vi "Main.vi"() -> ()   [LabVIEW 2023]
uses:
  UserCredentials.ctl
  Schedule.ctl
  stepvariables.ctl
  biasdiff.ctl
  gridvals.ctl
  remoterdgs.ctl
  QSM - Main/Controls/State Machine Message.ctl
  QSM - Main/Controls/Message Queue Element Position.ctl
  QSM - Main/QSM - Main.lvlib
panel:
  in  "Digital IO":bool[](array[boolean])
  in  "Analog IO":dbl[](array[numeric])
  in  "OffsetGain":dbl[](array[numeric])
  out "remrdgs":T1
  in  "Param Gx Only":cluster{"P06 G1 ONLY":bool, "P21 G2 ONLY":bool}
  in  "GXVALS":T2
  in  "BIAS DIFF":T3 {"DIFF" step=10.0; "BIAS" step=10.0}
  out "LIMITS":sgl[](array[numeric])
  out "Run Results":i32[](listbox)
  out "ALARM":bool
  out "PROC NOK":bool
  in  "ALARMS":bool[](array[boolean])=[FALSE]
  in  "PROC OK":bool[](array[boolean])=[TRUE]
  out "STEP VARS":T4
  in  "PLC CURRENT STEP":u16
  in  "RESET Button":bool
  in  "RUN Button":bool
  in  "FINAL STEP":u16
  out "CURRENT STEP":u16
  in  "FIRST STEP":u16
  in  "ALARMS BUtton":bool
  in  "LIMITS Button":bool
  in  "IO/DOCS Button":bool
  in  "ENTER OP":string
  in  "ENTER SN":string
  in  "View Sched Button":bool
  in  "Schedule":T5 caption="Multicolumn Listbox"
  out "SchedNames[]":string[](array[string])
  out "SchedName":string
  out "SchedNum":string
  in  "sched sel Button":bool
  out "schd61-80":u32
  out "schd31-60":u32
  out "schd1-30":u32
  out "AP%":dbl
  out "T10":dbl
  out "T100":dbl
  out "HS":dbl
  out "RTC":dbl
  out "NAME":string
  out "TUBE":dbl
  in  "Load Tube Button":bool
  in  "Error In":errorcluster
  out "Error Out":errorcluster
  in  "Security Button":bool
  in  "stop":bool
  out "Access":u16
  out "Op Name":string
  out "BADGE NUMBER":string
  in  "Log In Button":bool
  in  "Editor Button":bool
  in  "User Creds":T6
  # "--STEP VARIABLES--"
  # "--GRID TANK VALUES--"
  # "--CONTROLS--"
  # "ENTER SN"
  # "ENTER OP"
  # "--READINGS--"
  # "FOCAL SPOT GRID TANK RUN RESULTS"
  # "OFFSET"
  # "GAIN"
  # "OFFSET"
  # "GAIN"
  # "GAIN"
  # "OFFSET"
  # "GAIN"
  # "STEP"
  # "NAME"
  # "NOTES"
  # "PARAMS"
  # "KV SP"
  # "KV RDG"
  # "MA/IF SP"
  # "MA/IF RDG"
  # "EXP sec SP"
  # "EXP sec RDG"
  # "COOL sec SP"
  # "COOL sec RDG"
  # "scans.Mode"
  # "data item"
  # "min"
  # "max"
  # "init BIAS SP"
  # "init BIAS RDG"
  # "init DIFF SP"
  # "max Gx"
  # "init EfDr SP"
  # "init EfDr RDG"
  # "max Tries"
  # "TEST"
  # "LIM1"
  # "LIM2"
  # "LIM4"
  # "LIM3"
  # "CHAIN SCHEDS"
  # "RPTS"
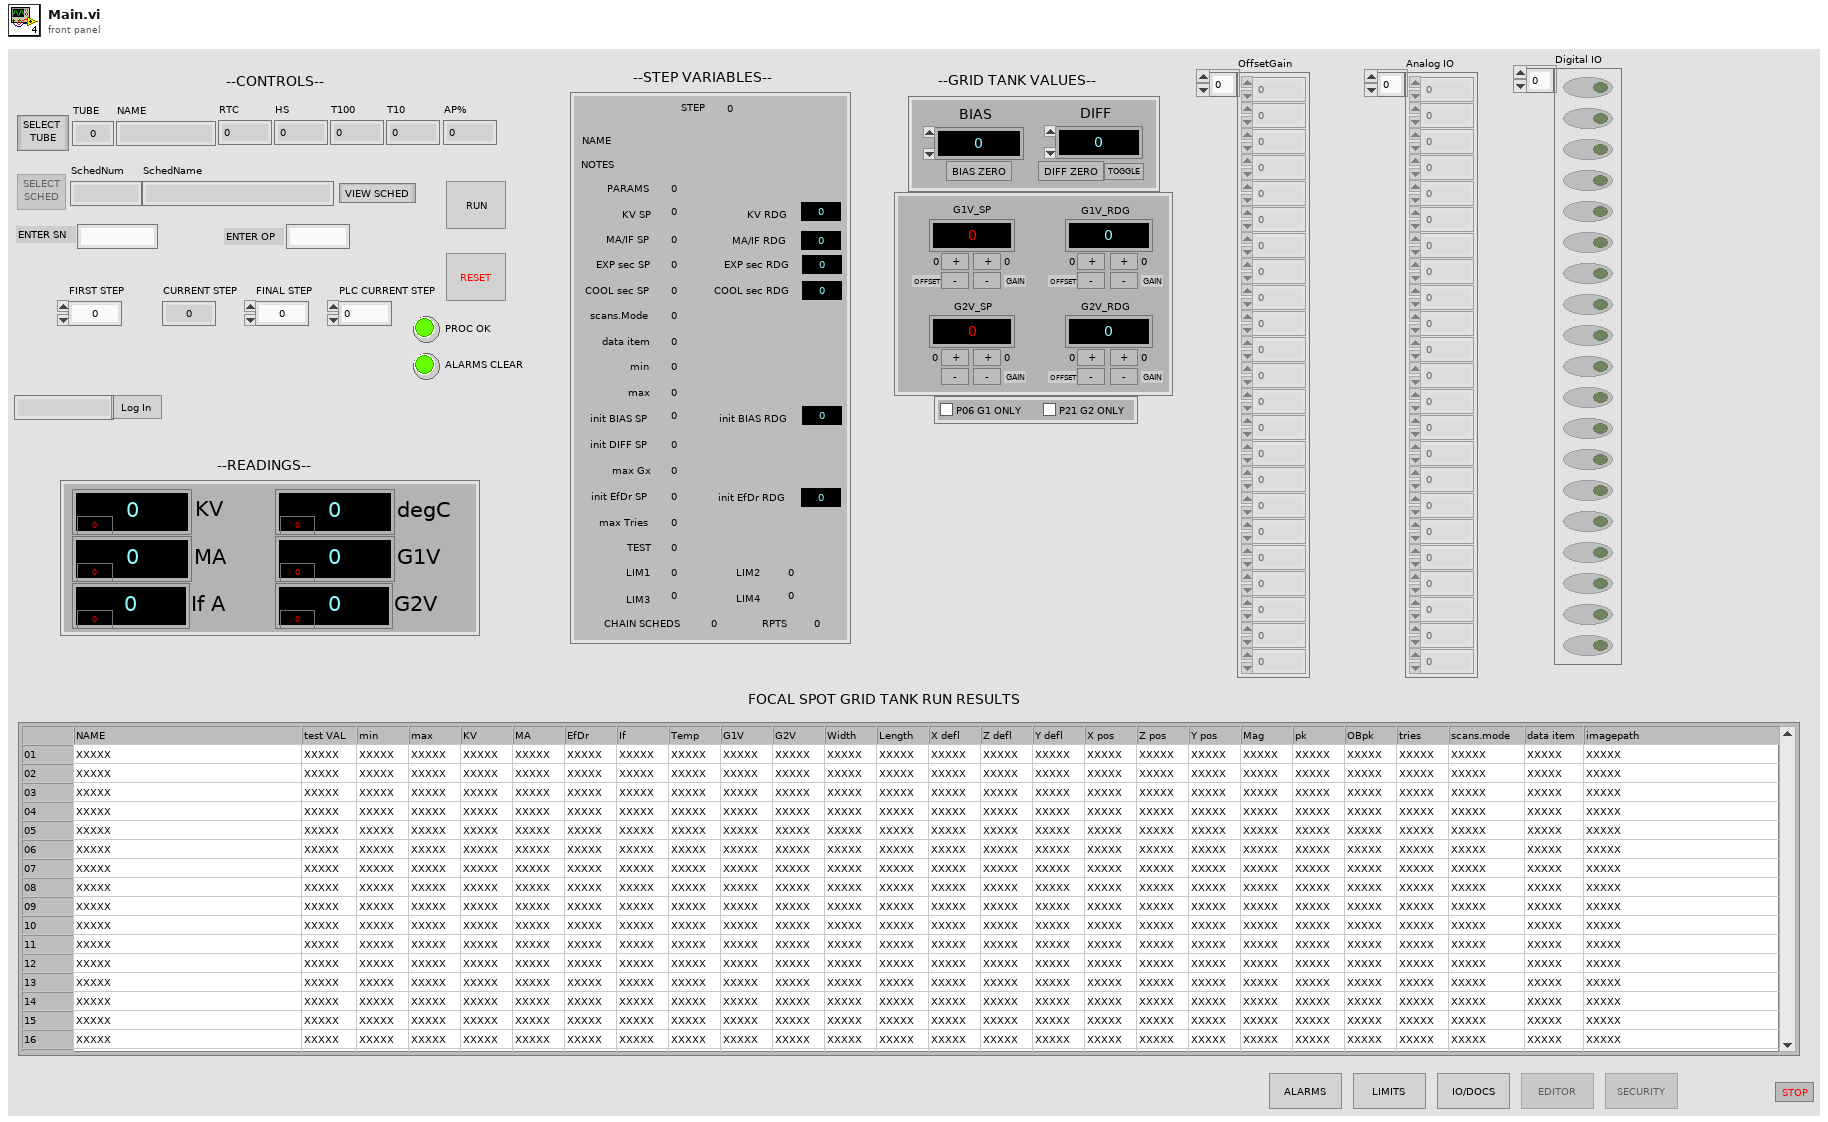
[diagram p1: front panel]
types:
  T1 = typedef "remoterdgs.ctl" = cluster{"remKVrdg":dbl, "remMArdg":dbl, "remIfArdg":dbl, "Temprdg":dbl, "G1Vrdg":dbl, "G2Vrdg":dbl, "remKVsp":dbl, "remMAsp":dbl, "remIfAsp":dbl, "Tempsp":dbl, "G1Vsp":dbl, "G2Vsp":dbl}
  T2 = typedef "gridvals.ctl" = cluster{"G1V_SP":dbl, "G2V_SP":dbl, "G1V_RDG":dbl, "G2V_RDG":dbl, "G1sp offset up":bool, "G1sp offset down":bool, "G1sp gain up":bool, "G1sp gain down":bool, "G1rdg offset up":bool, "G1rdg offset down":bool, "G1rdg gain up":bool, "G1rdg gain down":bool, "G2sp offset up":bool, "G2sp offset down":bool, "G2sp gain up":bool, "G2sp gain down":bool, "G2rdg offset up":bool, "G2rdg offset down":bool, "G2rdg gain up":bool, "G2rdg gain down":bool, "g1spoffset":dbl, "g1spgain":dbl, "g2spoffset":dbl, "g2spgain":dbl, "g1rdgoffset":dbl, "g1rdggain":dbl, "g2rdgoffset":dbl, "g2rdggain":dbl}
  T3 = typedef "biasdiff.ctl" = cluster{"BIAS":dbl, "BIAS_ZER":bool, "BIAS_ZER 2":bool, "DIFF_TOGGLE":bool, "DIFF":dbl}
  T4 = typedef "stepvariables.ctl" = cluster{"NAME":string, "NOTES":string, "PARAMS":u32, "KV  SP":dbl, "KV  RDG":dbl, "MA/IF  SP":dbl, "MA/IF  RDG":dbl, "init BIAS SP":dbl, "init BIAS RDG":dbl, "max Gx":dbl, "TEST":u32, "min":dbl, "max":dbl, "LIM1":dbl, "LIM2":dbl, "LIM3":dbl, "LIM4":dbl, "data item":dbl, "chain scheds":dbl, "REPEATS":dbl, "STEP NUM":u32, "EXP s SP":dbl, "EXP s RDG":dbl, "COOL s SP":dbl, "COOL s RDG":dbl, "scans mode":dbl, "init EfDr":dbl, "init EfDr RDG":dbl, "max Tries":dbl, "init DIFF SP":dbl}
  T5 = typedef "Schedule.ctl" = i32
  T6 = typedef "UserCredentials.ctl" = cluster{"Badge Number":string, "Name":string, "Access":enum16{"", "Operator", "Admin", "Engineer"}}
  T7 = typedef "QSM - Main.lvlib/State Machine Message.ctl" = enum16{"Initialize", "Operator Signon", "Editor", "Security", "Select Tube", "Select Sched", "View Sched", "View IO/DOCS", "View LIMITS", "View ALARMS", "Start Step Change", "New Serial Number", "RUN Initiated", "RESET Initiated", "PLC Step Change", "PROC OK CHECK", "PROC NOK", "ALARM CHECK", "ALARM ACTIVE", "Handle Error", "Exit"}
  T8 = typedef "QSM - Main.lvlib/Message Queue Element Position.ctl" = enum16{"Front", "Back"}
  T9 = enum8{"Enabled", "Disabled", "Disabled and Grayed Out"}
  T10 = typedef "UserCredentials.ctl" = cluster{"Badge Number":string, "Name":string, "Access":u16}
  T11 = cluster{"NO GRID TANK":bool, "NO GRID TANK 2":bool, "NO GRID TANK 3":bool, "NO GRID TANK 4":bool, "NO GRID TANK 5":bool, "NO GRID TANK 6":bool, "NO GRID TANK 7":bool, "NO GRID TANK 8":bool}
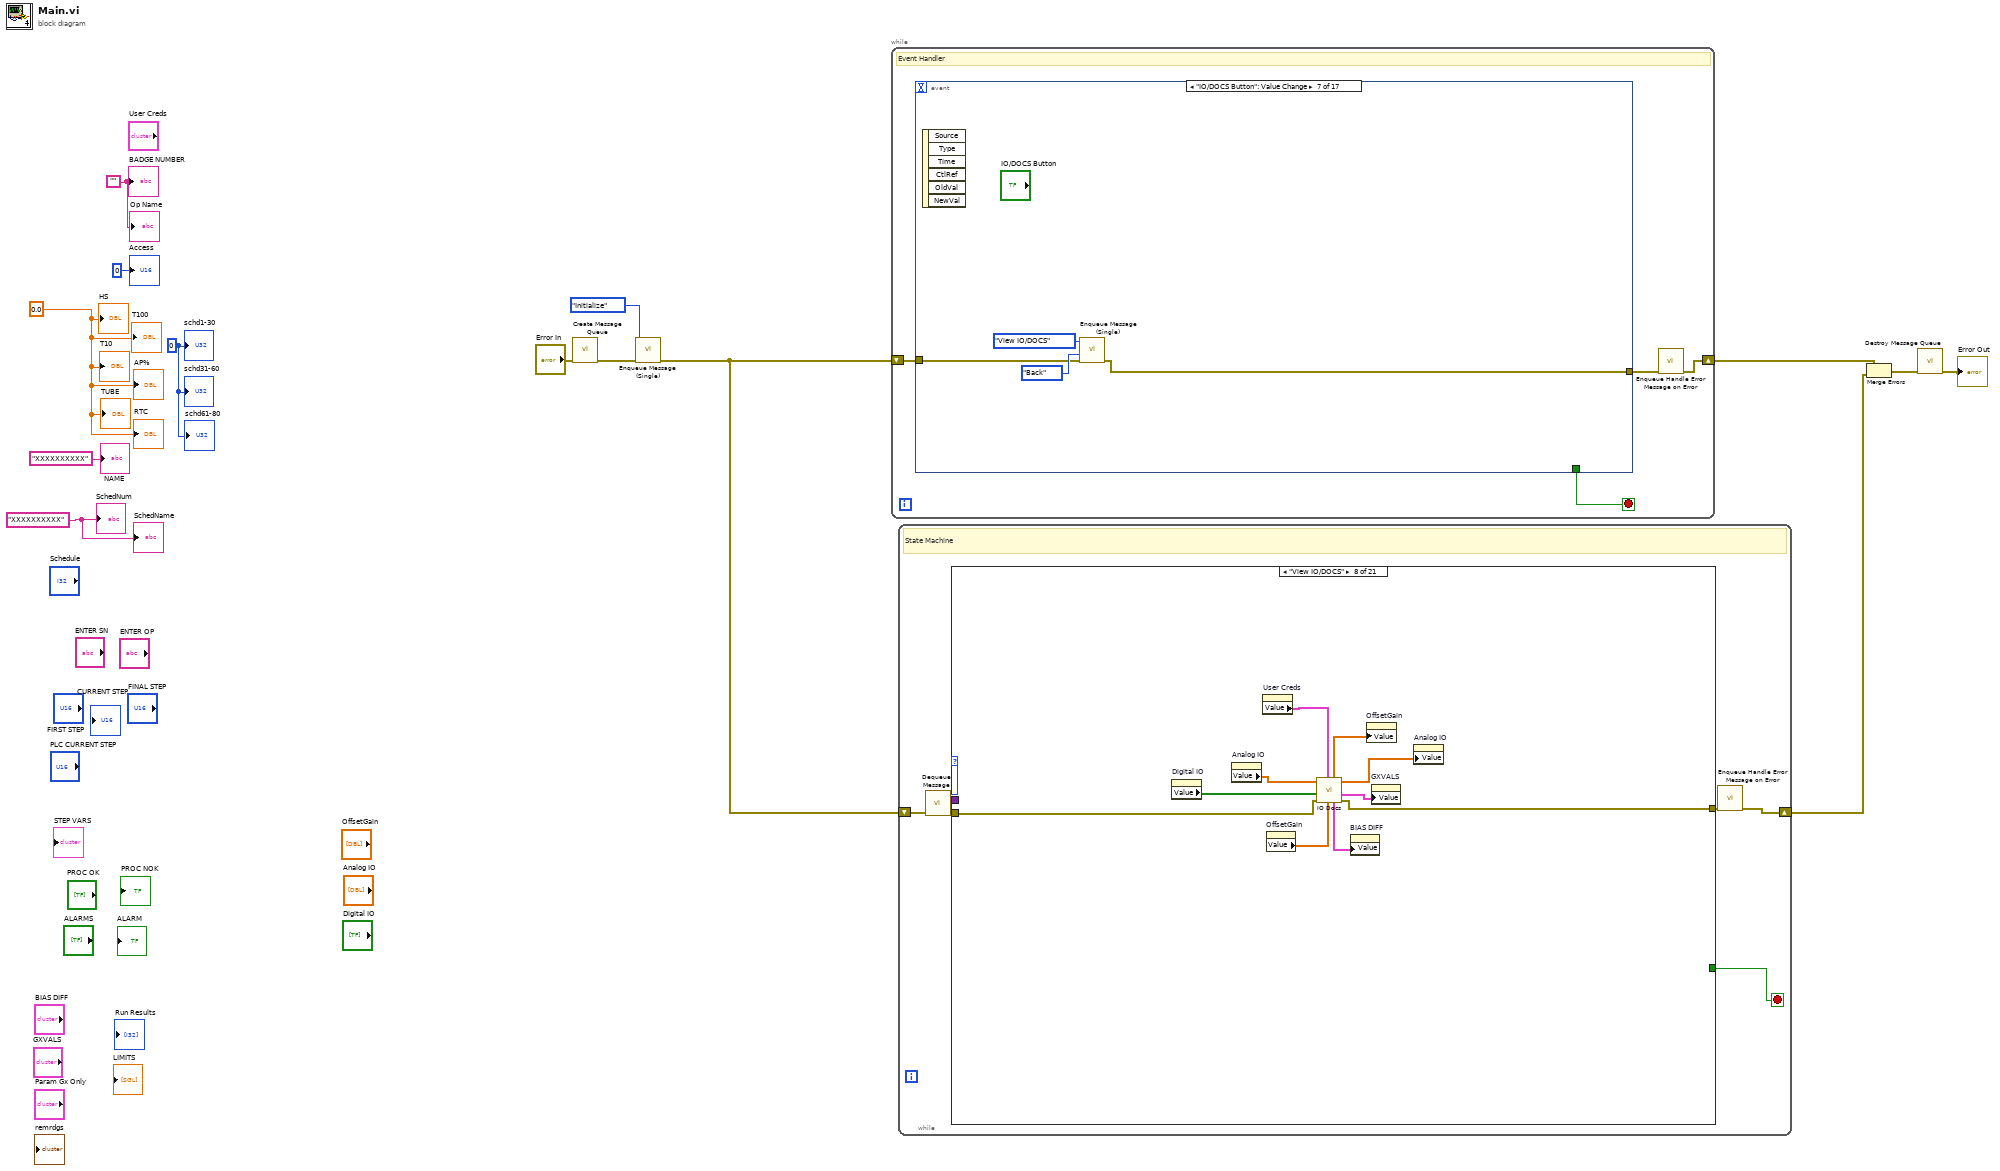
[diagram p0: block diagram]
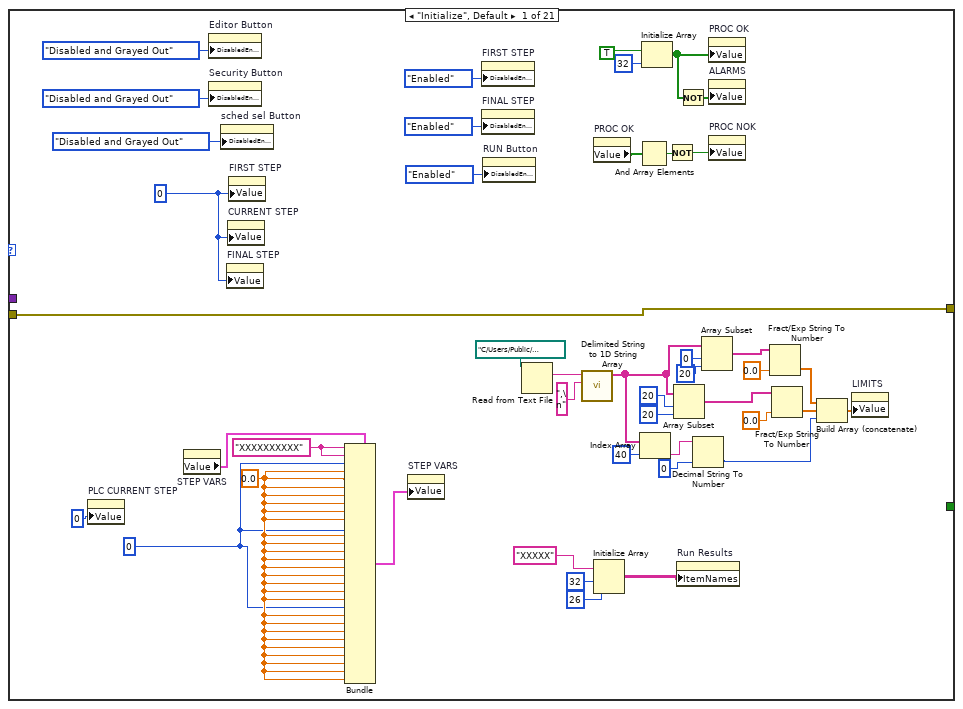
[diagram p2: hidden frame]
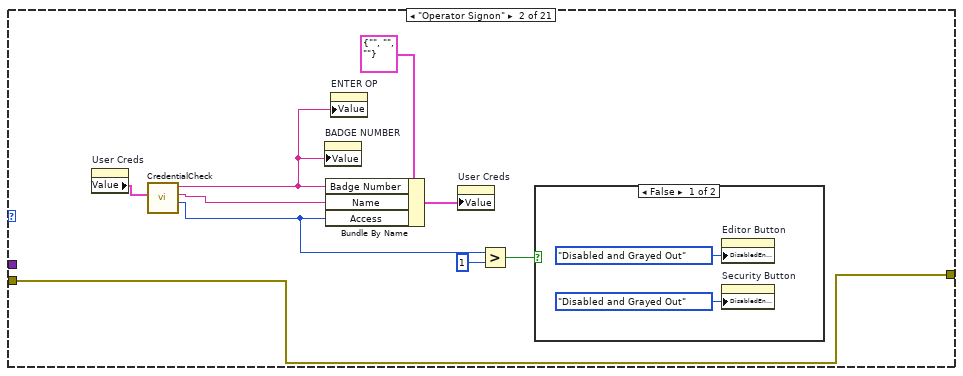
[diagram p3: hidden frame]
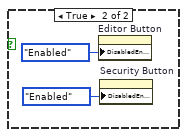
[diagram p4: hidden frame]
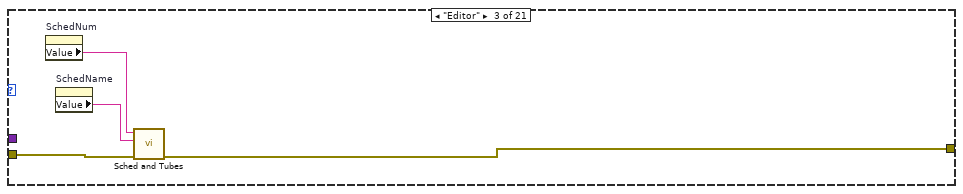
[diagram p5: hidden frame]
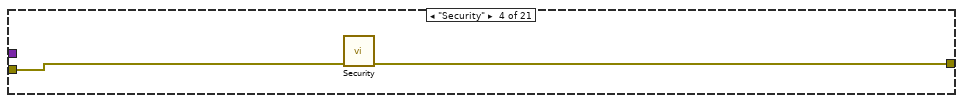
[diagram p6: hidden frame]
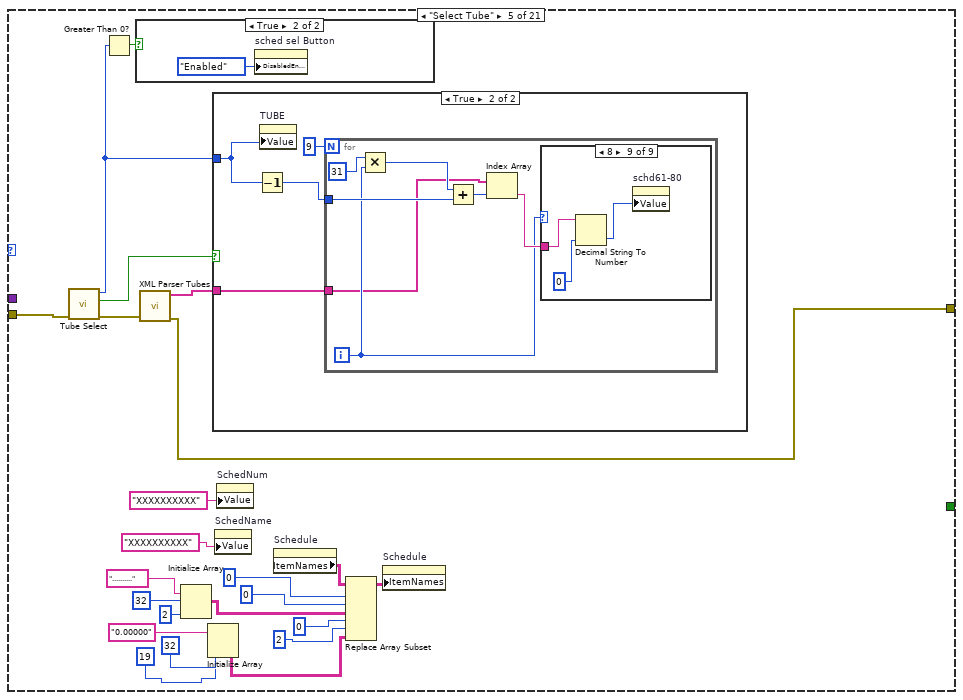
[diagram p7: hidden frame]
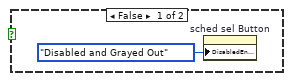
[diagram p8: hidden frame]
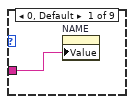
[diagram p10: hidden frame]
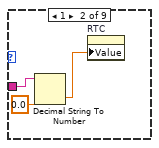
[diagram p11: hidden frame]
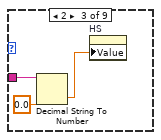
[diagram p12: hidden frame]
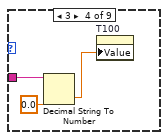
[diagram p13: hidden frame]
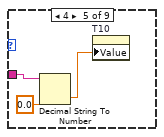
[diagram p14: hidden frame]
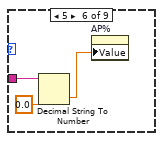
[diagram p15: hidden frame]
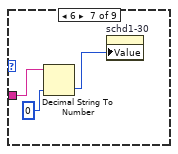
[diagram p16: hidden frame]
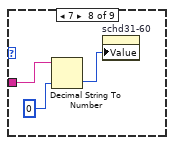
[diagram p17: hidden frame]
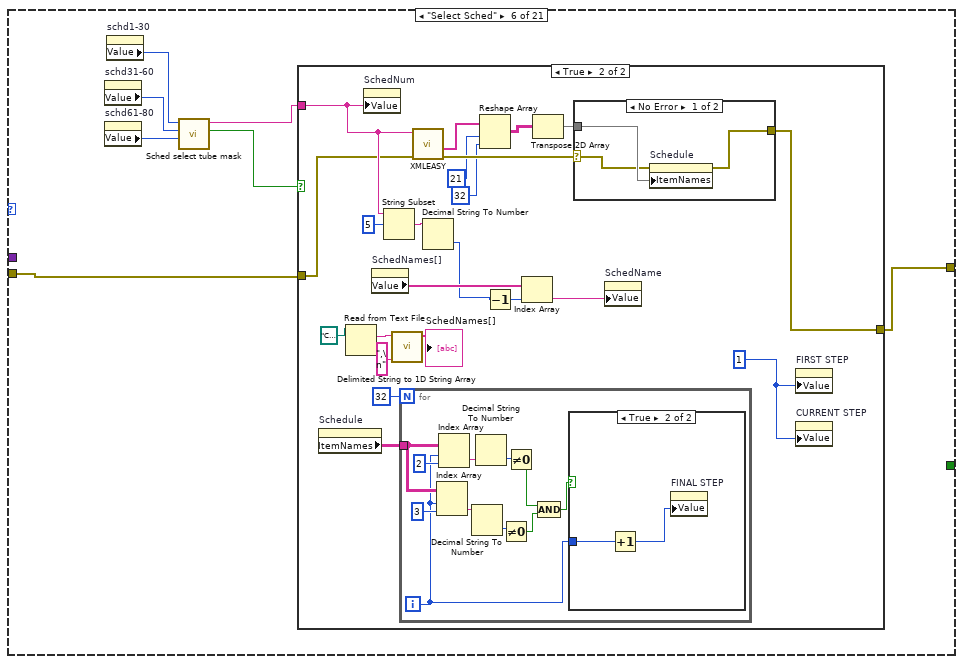
[diagram p18: hidden frame]
diagram:
  w1 = "XXXXXXXXXX" ("SchedNum")
  w2 = u32 0 ("schd1-30")
  w3 = 0.0 ("HS")
  w14 = "" ("Badge Number")
  n1 = call "Create Message Queue.vi"("Error In"="Error In") -> ("Error Out"=w12:errorcluster)  [unwired: 10 in]
  n2 = call "Enqueue Message (Single).vi"("Error In"=w12, "State Machine Message"=State_Machine_Message."Initialize") -> ("Error Out"=w6:errorcluster)  [unwired: 9 in]
  n3 = while {
    shift-right: [w15] -> w10
    shift-left: w6 -> [w17]
    stop <- w18 stop-if-true
    # "Event Handler"
    n4 = event shown="[6] \"IO/DOCS Button\": Value Change" {
      selector: _ -> [_ _ _ _ _ _ _ _ _ _ _ _ _ _ _ _ _]
      dyn-events: _ -> [_ _ _ _ _ _ _ _ _ _ _ _ _ _ _ _ _]
      timeout: _ -> [_ _ _ _ _ _ _ _ _ _ _ _ _ _ _ _ _]
      tunnel: [_ _ _ _ _ _ _ _ _ _ _ _ _ _ _ _ TRUE] -> w18
      tunnel: w17 -> [w20 w24 w30 w32 w36 w40 w44 w48 w52 w56 w60 w64 w68 w72 w76 w80 w84]
      tunnel: [w19 w23 w29 w31 w35 w39 w43 w47 w51 w55 w59 w63 w67 w71 w75 w79 w83] -> w16
      event "Log In Button": Value Change {
        n5 = event-data() -> ()  [unwired: 1 in, 6 out]
        n6 = call "Enqueue Message (Single).vi"("Error In"=w20, "Message Position"=Message_Queue_Element_Position."Back", "State Machine Message"=State_Machine_Message."Operator Signon") -> ("Error Out"=w19:errorcluster)  [unwired: 8 in]
      }
      event "Editor Button": Value Change {
        n7 = event-data() -> ()  [unwired: 1 in, 6 out]
        n8 = call "Enqueue Message (Single).vi"("Error In"=w24, "Message Position"=Message_Queue_Element_Position."Back", "State Machine Message"=State_Machine_Message."Editor") -> ("Error Out"=w23:errorcluster)  [unwired: 8 in]
      }
      event "Security Button": Value Change {
        n9 = event-data() -> ()  [unwired: 1 in, 6 out]
        n10 = call "Enqueue Message (Single).vi"("Error In"=w30, "Message Position"=Message_Queue_Element_Position."Back", "State Machine Message"=State_Machine_Message."Security") -> ("Error Out"=w29:errorcluster)  [unwired: 8 in]
      }
      event "Load Tube Button": Value Change {
        n11 = event-data() -> ()  [unwired: 1 in, 6 out]
        n12 = call "Enqueue Message (Single).vi"("Error In"=w32, "Message Position"=Message_Queue_Element_Position."Back", "State Machine Message"=State_Machine_Message."Select Tube") -> ("Error Out"=w31:errorcluster)  [unwired: 8 in]
      }
      event "sched sel Button": Value Change {
        n13 = event-data() -> ()  [unwired: 1 in, 6 out]
        n14 = call "Enqueue Message (Single).vi"("Error In"=w36, "Message Position"=Message_Queue_Element_Position."Back", "State Machine Message"=State_Machine_Message."Select Sched") -> ("Error Out"=w35:errorcluster)  [unwired: 8 in]
      }
      event "View Sched Button": Value Change {
        n15 = event-data() -> ()  [unwired: 1 in, 6 out]
        n16 = call "Enqueue Message (Single).vi"("Error In"=w40, "Message Position"=Message_Queue_Element_Position."Back", "State Machine Message"=State_Machine_Message."View Sched") -> ("Error Out"=w39:errorcluster)  [unwired: 8 in]
      }
      event "IO/DOCS Button": Value Change {
        n17 = event-data() -> ()  [unwired: 1 in, 6 out]
        n18 = call "Enqueue Message (Single).vi"("Error In"=w44, "Message Position"=Message_Queue_Element_Position."Back", "State Machine Message"=State_Machine_Message."View IO/DOCS") -> ("Error Out"=w43:errorcluster)  [unwired: 8 in]
      }
      event "LIMITS Button": Value Change {
        n19 = event-data() -> ()  [unwired: 1 in, 6 out]
        n20 = call "Enqueue Message (Single).vi"("Error In"=w48, "Message Position"=Message_Queue_Element_Position."Back", "State Machine Message"=State_Machine_Message."View LIMITS") -> ("Error Out"=w47:errorcluster)  [unwired: 8 in]
      }
      event "ALARMS BUtton": Value Change {
        n21 = event-data() -> ()  [unwired: 1 in, 6 out]
        n22 = call "Enqueue Message (Single).vi"("Error In"=w52, "Message Position"=Message_Queue_Element_Position."Back", "State Machine Message"=State_Machine_Message."View ALARMS") -> ("Error Out"=w51:errorcluster)  [unwired: 8 in]
      }
      event "FIRST STEP": Value Change {
        n23 = event-data() -> ()  [unwired: 1 in, 6 out]
        n24 = call "Enqueue Message (Single).vi"("Error In"=w56, "Message Position"=Message_Queue_Element_Position."Back", "State Machine Message"=State_Machine_Message."Start Step Change") -> ("Error Out"=w55:errorcluster)  [unwired: 8 in]
      }
      event "PLC CURRENT STEP": Value Change {
        n25 = event-data() -> ()  [unwired: 1 in, 6 out]
        n26 = call "Enqueue Message (Single).vi"("Error In"=w60, "Message Position"=Message_Queue_Element_Position."Back", "State Machine Message"=State_Machine_Message."PLC Step Change") -> ("Error Out"=w59:errorcluster)  [unwired: 8 in]
      }
      event "ENTER SN": Value Change {
        n27 = event-data() -> ()  [unwired: 1 in, 6 out]
        n28 = call "Enqueue Message (Single).vi"("Error In"=w64, "Message Position"=Message_Queue_Element_Position."Back", "State Machine Message"=State_Machine_Message."PLC Step Change") -> ("Error Out"=w63:errorcluster)  [unwired: 8 in]
      }
      event "RUN Button": Value Change {
        n29 = event-data() -> ()  [unwired: 1 in, 6 out]
        n30 = call "Enqueue Message (Single).vi"("Error In"=w68, "Message Position"=Message_Queue_Element_Position."Back", "State Machine Message"=State_Machine_Message."RUN Initiated") -> ("Error Out"=w67:errorcluster)  [unwired: 8 in]
      }
      event "RESET Button": Value Change {
        n31 = event-data() -> ()  [unwired: 1 in, 6 out]
        n32 = call "Enqueue Message (Single).vi"("Error In"=w72, "Message Position"=Message_Queue_Element_Position."Back", "State Machine Message"=State_Machine_Message."RESET Initiated") -> ("Error Out"=w71:errorcluster)  [unwired: 8 in]
      }
      event "PROC OK": Value Change {
        n33 = event-data() -> ()  [unwired: 1 in, 6 out]
        n34 = call "Enqueue Message (Single).vi"("Error In"=w76, "Message Position"=Message_Queue_Element_Position."Front", "State Machine Message"=State_Machine_Message."PROC OK CHECK") -> ("Error Out"=w75:errorcluster)  [unwired: 8 in]
      }
      event "ALARMS": Value Change {
        n35 = event-data() -> ()  [unwired: 1 in, 6 out]
        n36 = call "Enqueue Message (Single).vi"("Error In"=w80, "Message Position"=Message_Queue_Element_Position."Front", "State Machine Message"=State_Machine_Message."ALARM CHECK") -> ("Error Out"=w79:errorcluster)  [unwired: 8 in]
      }
      event "stop": Value Change {
        n37 = event-data() -> ()  [unwired: 1 in, 6 out]
        n38 = call "Enqueue Message (Single).vi"("Error In"=w84, "Message Position"=Message_Queue_Element_Position."Front", "State Machine Message"=State_Machine_Message."Exit") -> ("Error Out"=w83:errorcluster)  [unwired: 8 in]
      }
    }
    n39 = call "Enqueue Handle Error Message on Error.vi"("Error In"=w16) -> ("Error Out"=w15:errorcluster)  [unwired: 10 in]
  }
  n40 = while {
    shift-right: [w90] -> w9
    shift-left: w6 -> [w88]
    stop <- w89 stop-if-true
    # "State Machine"
    n41 = call "Dequeue Message.vi"("Error In"=w88) -> ("Error Out"=w92:errorcluster, "Data"=w93:variant, "State Machine Message"=w94:T7)  [unwired: 8 in]
    n42 = case shown="\"View IO/DOCS\"" w94 {
      tunnel: w93 -> [_ _ _ _ _ _ _ _ _ _ _ _ _ _ _ _ _ _ _ w371 _]
      tunnel: w92 -> [w115 w141 w155 w157 w180 w220 w269 w279 w288 w297 w300 w302 w304 w332 w338 w344 w355 w358 w366 w369 w374]
      tunnel: [w115 w141 w154 w156 w176 w219 w269 w278 w287 w296 w298 w302 w304 w332 w338 w343 w355 w357 w366 w367 w373] -> w91
      tunnel: [_ _ _ _ _ _ _ _ _ _ _ _ _ _ _ _ _ _ _ _ TRUE] -> w89
      frame "Initialize", Default {
        w95 = u32 0 ("PARAMS")
        w130 = 0.0
        w131 = "XXXXXXXXXX" ("NAME")
        w135 = 0 ("STARTING STEP")
        n43 = property on="PLC CURRENT STEP" class="DigNum (strict)"("Value"=u16 0 ("PLC CURRENT STEP 2")) -> ()  [unwired: 2 in, 2 out]
        n44 = property on="STEP VARS" class="Clust (strict)"() -> ("Value"=w132:T4)  [unwired: 2 in, 2 out]
        n45 = property on="Editor Button" class="Bool"("DisabledEnum"=T9."Disabled and Grayed Out" ("Disabled")) -> ()  [unwired: 2 in, 2 out]
        n46 = property on="Security Button" class="Bool (strict)"("DisabledEnum"=T9."Disabled and Grayed Out" ("Disabled")) -> ()  [unwired: 2 in, 2 out]
        n47 = property on="sched sel Button" class="Bool (strict)"("DisabledEnum"=T9."Disabled and Grayed Out" ("Disabled")) -> ()  [unwired: 2 in, 2 out]
        n48 = property on="FINAL STEP" class="DigNum (strict)"("Value"=w135) -> ()  [unwired: 2 in, 2 out]
        n49 = property on="CURRENT STEP" class="DigNum (strict)"("Value"=w135) -> ()  [unwired: 2 in, 2 out]
        n50 = property on="FIRST STEP" class="DigNum (strict)"("Value"=w135) -> ()  [unwired: 2 in, 2 out]
        n51 = Bundle(cluster=w132, "NAME"=w131, "NOTES"=w131, "PARAMS"=w95, "KV  SP"=w130, "KV  RDG"=w130, "MA/IF  SP"=w130, "MA/IF  RDG"=w130, "init BIAS SP"=w130, "init BIAS RDG"=w130, "max Gx"=w130, "TEST"=w95, "min"=w130, "max"=w130, "LIM1"=w130, "LIM2"=w130, "LIM3"=w130, "LIM4"=w130, "data item"=w130, "chain scheds"=w130, "REPEATS"=w130, "STEP NUM"=w95, "EXP s SP"=w130, "EXP s RDG"=w130, "COOL s SP"=w130, "COOL s RDG"=w130, "scans mode"=w130, "init EfDr"=w130, "init EfDr RDG"=w130, "max Tries"=w130, "init DIFF SP"=w130) -> (w96:T4)
        n52 = property on="STEP VARS" class="Clust (strict)"("Value"=w96) -> ()  [unwired: 2 in, 2 out]
        n53 = property on="FIRST STEP" class="DigNum (strict)"("DisabledEnum"=T9."Enabled" ("Disabled")) -> ()  [unwired: 2 in, 2 out]
        n54 = property on="FINAL STEP" class="DigNum (strict)"("DisabledEnum"=T9."Enabled" ("Disabled")) -> ()  [unwired: 2 in, 2 out]
        n55 = property on="RUN Button" class="Bool (strict)"("DisabledEnum"=T9."Enabled" ("Disabled")) -> ()  [unwired: 2 in, 2 out]
        n56 = Read from Text File(file (use dialog)=path "C:/Users/Public/Documents/Grid2093/LIMITS/LIMITS.txt") -> (text=w110:string)  [unwired: 3 in, 3 out]
        n57 = call <vilib>:"Delimited String to 1D String Array.vi"("delimiter"=",\n", "delimited string"=w110) -> ("string array"=w113:string[])  [unwired: 9 in]
        n58 = property on="PROC OK" class="Arr (strict)"() -> ("Value"=w123:bool[])  [unwired: 2 in, 2 out]
        n59 = Initialize Array("XXXXX", 32 ("dimension size"), 26 ("dimension size")) -> (w117:string[][])
        n60 = And Array Elements(Boolean array=w123) -> (logical AND=w122:bool)
        n61 = Index Array(array=w113, index=40) -> (element=w114:string)
        n62 = Initialize Array(TRUE, 32 ("dimension size")) -> (w125:bool[])
        n63 = Not(x=w122) -> (.not. x?=w121:bool)
        n64 = Array Subset(array=w113, index=20, length=20) -> (w112:string[])
        n65 = property on="Run Results" class="MCListbox (strict)"("ItemNames"=w117) -> ()  [unwired: 2 in, 2 out]
        n66 = Not(x=w125) -> (.not. x?=w124:bool[])
        n67 = Decimal String To Number(string=w114, default (0L)=u32 0 ("default (0 I32)")) -> (number=w97:u32)  [unwired: 1 in, 1 out]
        n68 = Array Subset(array=w113, index=0, length=20) -> (w111:string[])
        n69 = property on="PROC OK" class="Arr (strict)"("Value"=w125) -> ()  [unwired: 2 in, 2 out]
        n70 = property on="ALARMS" class="Arr (strict)"("Value"=w124) -> ()  [unwired: 2 in, 2 out]
        n71 = property on="PROC NOK" class="Bool (strict)"("Value"=w121) -> ()  [unwired: 2 in, 2 out]
        n72 = Fract/Exp String To Number(string=w111, default (0 dbl)=sgl 0.0 ("default (0 DBL)")) -> (number=w99:sgl[])  [unwired: 2 in, 1 out]
        n73 = Fract/Exp String To Number(string=w112, default (0 dbl)=sgl 0.0 ("default (0 DBL)")) -> (number=w98:sgl[])  [unwired: 2 in, 1 out]
        n74 = Build Array (concatenate)(w99, w98, w97) -> (w116:sgl[])
        n75 = property on="LIMITS" class="Arr (strict)"("Value"=w116) -> ()  [unwired: 2 in, 2 out]
      }
      frame "Operator Signon" {
        n76 = property on="User Creds" class="Clust (strict)"() -> ("Value"=w139:T10)  [unwired: 2 in, 2 out]
        n77 = call "CredentialCheck.vi"("User Creds"=w139) -> ("Access"=w145:u16, "Name"=w144:string, "Badge Num"=w140:string)  [unwired: 8 in]
        n78 = property on="BADGE NUMBER" class="Str"("Value"=w140) -> ()  [unwired: 2 in, 2 out]
        n79 = Bundle By Name(cluster=T6 {"Badge Number"="", "Name"="", "Access"=enum.""} ("User Creds"), "Badge Number"=w140, "Name"=w144, "Access"=w145) -> (w143:T6)
        n80 = property on="ENTER OP" class="Str"("Value"=w140) -> ()  [unwired: 2 in, 2 out]
        n81 = property on="User Creds" class="Clust (strict)"("Value"=w143) -> ()  [unwired: 2 in, 2 out]
        n82 = Greater?(x=w145, y=u16 1) -> (0:w142:bool)
        n83 = case shown="False" w142 {
          frame False {
            n84 = property on="Editor Button" class="Bool"("DisabledEnum"=T9."Disabled and Grayed Out" ("Disabled")) -> ()  [unwired: 2 in, 2 out]
            n85 = property on="Security Button" class="Bool (strict)"("DisabledEnum"=T9."Disabled and Grayed Out" ("Disabled")) -> ()  [unwired: 2 in, 2 out]
          }
          frame True {
            n86 = property on="Editor Button" class="Bool"("DisabledEnum"=T9."Enabled" ("Disabled")) -> ()  [unwired: 2 in, 2 out]
            n87 = property on="Security Button" class="Bool (strict)"("DisabledEnum"=T9."Enabled" ("Disabled")) -> ()  [unwired: 2 in, 2 out]
          }
        }
      }
      frame "Editor" {
        n88 = property on="SchedNum" class="Str"() -> ("Value"=w153:string)  [unwired: 2 in, 2 out]
        n89 = property on="SchedName" class="Str"() -> ("Value"=w152:string)  [unwired: 2 in, 2 out]
        n90 = call "Sched and Tubes.vi"("Error In"=w155, "Preselected sched name"=w152, "Preselected sched"=w153) -> ("Error Out"=w154:errorcluster)  [unwired: 8 in]
      }
      frame "Security" {
        n91 = call "Security.vi"("Error In"=w157) -> ("error out"=w156:errorcluster)  [unwired: 10 in]
      }
      frame "Select Tube" {
        n92 = call "Tube Select.vi"("error in (no error)"=w180) -> ("error out"=w178:errorcluster, "Load"=w179:bool, "SelectedTube"=w175:i32)  [unwired: 7 in, 1 out]
        n93 = Greater Than 0?(x=w175) -> (x > 0?=w174:bool)
        n94 = case shown="True" w174 {
          frame False {
            n95 = property on="sched sel Button" class="Bool (strict)"("DisabledEnum"=T9."Disabled and Grayed Out" ("Disabled")) -> ()  [unwired: 2 in, 2 out]
          }
          frame True {
            n96 = property on="sched sel Button" class="Bool (strict)"("DisabledEnum"=T9."Enabled" ("Disabled")) -> ()  [unwired: 2 in, 2 out]
          }
        }
        n97 = call "XML Parser Tubes.vi"("error in (no error)"=w178) -> ("error out"=w176:errorcluster, "output array"=w177:string[])  [unwired: 9 in]
        n98 = Initialize Array("..........", 32 ("dimension size"), 2 ("dimension size")) -> (w169:string[][])
        n99 = Initialize Array("0.00000", 32 ("dimension size"), 19 ("dimension size")) -> (w168:string[][])
        n100 = case shown="True" w179 {
          tunnel: w175 -> [_ w186]
          tunnel: w177 -> [_ w183]
          frame False {
          }
          frame True {
            n101 = Decrement(x=w186) -> (x-1=w184:i32)
            n102 = property on="TUBE" class="DigNum (strict)"("Value"=w186) -> ()  [unwired: 2 in, 2 out]
            n103 = for {
              N: 9 -> [_]
              tunnel: w184 -> [w191]
              tunnel: w183 -> [w187]
              i -> [w188]
              n104 = Multiply(x=31, y=w188) -> (x*y=w192:i32)
              n105 = Add(x=w192, y=w191) -> (x+y=w193:i32)
              n106 = Index Array(array=w187, index=w193) -> (element=w190:string)
              n107 = case shown="8" w188 {
                tunnel: w190 -> [w194 w197 w198 w201 w204 w207 w212 w214 w217]
                frame 0, Default {
                  n108 = property on="NAME" class="Str"("Value"=w194) -> ()  [unwired: 2 in, 2 out]
                }
                frame 1 {
                  n109 = Decimal String To Number(string=w197, default (0L)=0.0 ("RTC")) -> (number=w196:dbl)  [unwired: 1 in, 1 out]
                  n110 = property on="RTC" class="DigNum (strict)"("Value"=w196) -> ()  [unwired: 2 in, 2 out]
                }
                frame 2 {
                  n111 = Decimal String To Number(string=w198, default (0L)=0.0 ("RTC")) -> (number=w200:dbl)  [unwired: 1 in, 1 out]
                  n112 = property on="HS" class="DigNum (strict)"("Value"=w200) -> ()  [unwired: 2 in, 2 out]
                }
                frame 3 {
                  n113 = Decimal String To Number(string=w201, default (0L)=0.0 ("RTC")) -> (number=w203:dbl)  [unwired: 1 in, 1 out]
                  n114 = property on="T100" class="DigNum (strict)"("Value"=w203) -> ()  [unwired: 2 in, 2 out]
                }
                frame 4 {
                  n115 = Decimal String To Number(string=w204, default (0L)=0.0 ("RTC")) -> (number=w206:dbl)  [unwired: 1 in, 1 out]
                  n116 = property on="T10" class="DigNum (strict)"("Value"=w206) -> ()  [unwired: 2 in, 2 out]
                }
                frame 5 {
                  n117 = Decimal String To Number(string=w207, default (0L)=0.0 ("RTC")) -> (number=w209:dbl)  [unwired: 1 in, 1 out]
                  n118 = property on="AP%" class="DigNum (strict)"("Value"=w209) -> ()  [unwired: 2 in, 2 out]
                }
                frame 6 {
                  n119 = Decimal String To Number(string=w212, default (0L)=u32 0 ("default (0 I32)")) -> (number=w210:u32)  [unwired: 1 in, 1 out]
                  n120 = property on="schd1-30" class="DigNum (strict)"("Value"=w210) -> ()  [unwired: 2 in, 2 out]
                }
                frame 7 {
                  n121 = Decimal String To Number(string=w214, default (0L)=u32 0 ("default (0 I32)")) -> (number=w213:u32)  [unwired: 1 in, 1 out]
                  n122 = property on="schd31-60" class="DigNum (strict)"("Value"=w213) -> ()  [unwired: 2 in, 2 out]
                }
                frame 8 {
                  n123 = Decimal String To Number(string=w217, default (0L)=u32 0 ("default (0 I32)")) -> (number=w216:u32)  [unwired: 1 in, 1 out]
                  n124 = property on="schd61-80" class="DigNum (strict)"("Value"=w216) -> ()  [unwired: 2 in, 2 out]
                }
              }
            }
          }
        }
        n125 = property on="SchedName" class="Str"("Value"="XXXXXXXXXX" ("SchedNum")) -> ()  [unwired: 2 in, 2 out]
        n126 = property on="SchedNum" class="Str"("Value"="XXXXXXXXXX" ("SchedNum")) -> ()  [unwired: 2 in, 2 out]
        n127 = property on="Schedule" class="MCListbox (strict)"() -> ("ItemNames"=w171:string[][])  [unwired: 2 in, 2 out]
        n128 = Replace Array Subset(array=w171, new element #1=w169, index (row) #1=0 ("index"), index (col) #1=0 ("disabled index (col)"), new element #2=w168, index (row) #2=0 ("index"), index (col) #2=2 ("disabled index (col)")) -> (w170:string[][])
        n129 = property on="Schedule" class="MCListbox (strict)"("ItemNames"=w170) -> ()  [unwired: 2 in, 2 out]
      }
      frame "Select Sched" {
        n130 = property on="schd31-60" class="DigNum (strict)"() -> ("Value"=w224:u32)  [unwired: 2 in, 2 out]
        n131 = property on="schd61-80" class="DigNum (strict)"() -> ("Value"=w223:u32)  [unwired: 2 in, 2 out]
        n132 = property on="schd1-30" class="DigNum (strict)"() -> ("Value"=w225:u32)  [unwired: 2 in, 2 out]
        n133 = call "Sched select tube mask.vi"("sched61-80mask"=w223, "sched31-60mask"=w224, "sched1-30mask"=w225) -> ("Load"=w221:bool, "selected sched"=w222:string)  [unwired: 6 in, 1 out]
        n134 = case shown="True" w221 {
          tunnel: w222 -> [_ w248]
          tunnel: [w226 w231] -> w219
          tunnel: w220 -> [w226 w230]
          frame False {
          }
          frame True {
            w228 = u16 1 ("STARTING STEP")
            n135 = property on="Schedule" class="MCListbox (strict)"() -> ("ItemNames"=w227:string[][])  [unwired: 2 in, 2 out]
            n136 = Read from Text File(file (use dialog)=path "C:/Users/Public/Documents/Grid2093/SCHEDS/SchedNames.txt" ("path")) -> (text=w234:string)  [unwired: 3 in, 3 out]
            n137 = property on="SchedNum" class="Str"("Value"=w248) -> ()  [unwired: 2 in, 2 out]
            n138 = property on="SchedNames[]" class="Arr (strict)"() -> ("Value"=w239:string[])  [unwired: 2 in, 2 out]
            n139 = String Subset(string=w248, offset (0)=5) -> (substring=w241:string)  [unwired: 1 in]
            n140 = call <vilib>:"Delimited String to 1D String Array.vi"("delimiter"=",\n", "delimited string"=w234) -> ("string array"=→"SchedNames[]":string[])  [unwired: 9 in]
            n141 = for {
              N: 32 -> [_]
              tunnel: w227 -> [w256]
              i -> [w255]
              n142 = Index Array(array=w256, index (row)=w255, index (col)=3 ("disabled index (col)")) -> (element=w252:string)
              n143 = Index Array(array=w256, index (row)=w255, index (col)=2 ("disabled index (col)")) -> (element=w254:string)
              n144 = Decimal String To Number(string=w252) -> (number=w251:i32)  [unwired: 2 in, 1 out]
              n145 = Decimal String To Number(string=w254) -> (number=w253:i32)  [unwired: 2 in, 1 out]
              n146 = Not Equal To 0?(x=w251) -> (x != 0?=w250:bool)
              n147 = Not Equal To 0?(x=w253) -> (x != 0?=w249:bool)
              n148 = Compound Arithmetic op=AND(w249, w250) -> (w258:bool)
              n149 = case shown="True" w258 {
                tunnel: w255 -> [_ w261]
                frame False {
                }
                frame True {
                  n150 = Increment(x=w261) -> (x+1=w260:i32)
                  n151 = property on="FINAL STEP" class="DigNum (strict)"("Value"=w260) -> ()  [unwired: 2 in, 2 out]
                }
              }
            }
            n152 = call "XMLEASY.vi"("error in (no error)"=w230, "Schedule Filename"=w248) -> ("error out"=w247:errorcluster, "Sched Tag Vals (1D)"=w244:string[])  [unwired: 6 in, 2 out]
            n153 = Decimal String To Number(string=w241) -> (number=w236:i32)  [unwired: 2 in, 1 out]
            n154 = Reshape Array(w244, 21 ("dimension size"), 32 ("dimension size")) -> (w243:string[][])
            n155 = Decrement(x=w236) -> (x-1=w237:i32)
            n156 = Index Array(array=w239, index=w237) -> (element=w238:string)
            n157 = Transpose 2D Array(2D array=w243) -> (transposed array=w242:string[][])
            n158 = case shown="No Error" w247 {
              selector: w247 -> [w263 w265]
              tunnel: [w262 w265] -> w231
              tunnel: w242 -> [w264 _]
              frame No Error {
                n159 = property on="Schedule" class="MCListbox (strict)"(error in=w263, "ItemNames"=w264) -> (error out=w262:errorcluster)  [unwired: 1 in, 1 out]
              }
              frame Error {
              }
            }
            n160 = property on="SchedName" class="Str"("Value"=w238) -> ()  [unwired: 2 in, 2 out]
            n161 = property on="FIRST STEP" class="DigNum (strict)"("Value"=w228) -> ()  [unwired: 2 in, 2 out]
            n162 = property on="CURRENT STEP" class="DigNum (strict)"("Value"=w228) -> ()  [unwired: 2 in, 2 out]
          }
        }
      }
      frame "View Sched" {
        n163 = property on="Schedule" class="MCListbox (strict)"() -> ("ItemNames"=w268:string[][])  [unwired: 2 in, 2 out]
        n164 = property on="SchedName" class="Str"() -> ("Value"=w266:string)  [unwired: 2 in, 2 out]
        n165 = property on="SchedNum" class="Str"() -> ("Value"=w267:string)  [unwired: 2 in, 2 out]
        n166 = call "SchedViewOnly.vi"("schedname"=w266, "schednum"=w267, "SchedArray"=w268) -> ()  [unwired: 9 in]
      }
      frame "View IO/DOCS" {
        n167 = property on="Digital IO" class="Arr (strict)"() -> ("Value"=w271:bool[])  [unwired: 2 in, 2 out]
        n168 = property on="Analog IO" class="Arr (strict)"() -> ("Value"=w272:dbl[])  [unwired: 2 in, 2 out]
        n169 = property on="User Creds" class="Clust (strict)"() -> ("Value"=w270:T6)  [unwired: 2 in, 2 out]
        n170 = property on="OffsetGain" class="Arr (strict)"() -> ("Value"=w277:dbl[])  [unwired: 2 in, 2 out]
        n171 = call "IO Docs.vi"("OffsetGain"=w277, "User Creds"=w270, "Error In"=w279, "Digital IO"=w271, "Analog IO"=w272) -> ("Error Out"=w278:errorcluster, "GXVALS Output"=w275:T2, "Analog IO Out"=w273:dbl[], "BIAS DIFF Out"=w276:T3, "OffsetGain Out"=w274:dbl[])  [unwired: 2 in]
        n172 = property on="BIAS DIFF" class="Clust (strict)"("Value"=w276) -> ()  [unwired: 2 in, 2 out]
        n173 = property on="OffsetGain" class="Arr (strict)"("Value"=w274) -> ()  [unwired: 2 in, 2 out]
        n174 = property on="GXVALS" class="Clust (strict)"("Value"=w275) -> ()  [unwired: 2 in, 2 out]
        n175 = property on="Analog IO" class="Arr (strict)"("Value"=w273) -> ()  [unwired: 2 in, 2 out]
      }
      frame "View LIMITS" {
        n176 = call "LIMITS.vi"("Error In"=w288) -> ("Error Out"=w287:errorcluster, "Bool Lims Out"=w280:T11, "LIMITS Out"=w281:cluster{"LIMITS1-20":dbl[], "LIMITS21-40":dbl[]})  [unwired: 8 in]
        n177 = Cluster To Array(cluster=w280) -> (array=w286:bool[])
        n178 = Unbundle(w281) -> ("LIMITS1-20"=w285:dbl[], "LIMITS21-40"=w284:dbl[])
        n179 = Boolean Array To Number(Boolean array=w286) -> (number=w283:u32)
        n180 = Build Array (concatenate)(w285, w284, w283) -> (w282:dbl[])
        n181 = property on="LIMITS" class="Arr (strict)"("Value"=w282) -> ()  [unwired: 2 in, 2 out]
      }
      frame "View ALARMS" {
        n182 = property on="ALARMS" class="Arr (strict)"() -> ("Value"=w291:bool[])  [unwired: 2 in, 2 out]
        n183 = property on="PROC OK" class="Arr (strict)"() -> ("Value"=w295:bool[])  [unwired: 2 in, 2 out]
        n184 = call "ALARMS.vi"("Error In"=w297, "ALARM Input"=w291, "PROC OK Input"=w295) -> ("Error Out"=w296:errorcluster, "ALARM Output"=w290:bool[], "PROC OK Output"=w293:bool[])  [unwired: 6 in]
        n185 = Or Array Elements(Boolean array=w293) -> (logical OR=w292:bool)
        n186 = Not(x=w293) -> (.not. x?=w294:bool[])
        n187 = property on="PROC NOK" class="Bool (strict)"("Value"=w292) -> ()  [unwired: 2 in, 2 out]
        n188 = property on="PROC OK" class="Arr (strict)"("Value"=w294) -> ()  [unwired: 2 in, 2 out]
        n189 = Or Array Elements(Boolean array=w290) -> (logical OR=w289:bool)
        n190 = property on="ALARM" class="Bool (strict)"("Value"=w289) -> ()  [unwired: 2 in, 2 out]
        n191 = property on="ALARMS" class="Arr (strict)"("Value"=w290) -> ()  [unwired: 2 in, 2 out]
      }
      frame "Start Step Change" {
        n192 = property on="FIRST STEP" class="DigNum (strict)"(error in=w300) -> (error out=w299:errorcluster, "Value"=w301:u16)  [unwired: 1 in, 1 out]
        n193 = property on="CURRENT STEP" class="DigNum (strict)"(error in=w299, "Value"=w301) -> (error out=w298:errorcluster)  [unwired: 1 in, 1 out]
      }
      frame "New Serial Number" {
      }
      frame "RUN Initiated" {
        w303 = T9."Disabled and Grayed Out" ("Disabled")
        n194 = property on="FIRST STEP" class="DigNum (strict)"("DisabledEnum"=w303) -> ()  [unwired: 2 in, 2 out]
        n195 = property on="FINAL STEP" class="DigNum (strict)"("DisabledEnum"=w303) -> ()  [unwired: 2 in, 2 out]
        n196 = property on="RUN Button" class="Bool (strict)"("DisabledEnum"=w303) -> ()  [unwired: 2 in, 2 out]
        n197 = property on="Load Tube Button" class="Bool (strict)"("DisabledEnum"=w303) -> ()  [unwired: 2 in, 2 out]
        n198 = property on="sched sel Button" class="Bool (strict)"("DisabledEnum"=w303) -> ()  [unwired: 2 in, 2 out]
      }
      frame "RESET Initiated" {
        w307 = 0.0
        w308 = "XXXXXXXXXX" ("NAME")
        w314 = 0.0 ("RTC")
        n199 = property on="PLC CURRENT STEP" class="DigNum (strict)"("Value"=u16 0 ("PLC CURRENT STEP 2")) -> ()  [unwired: 2 in, 2 out]
        n200 = property on="FIRST STEP" class="DigNum (strict)"("DisabledEnum"=T9."Enabled" ("Disabled")) -> ()  [unwired: 2 in, 2 out]
        n201 = property on="FINAL STEP" class="DigNum (strict)"("DisabledEnum"=T9."Enabled" ("Disabled")) -> ()  [unwired: 2 in, 2 out]
        n202 = property on="NAME" class="Str"("Value"="XXXXXXXXXX" ("NAME")) -> ()  [unwired: 2 in, 2 out]
        n203 = property on="RUN Button" class="Bool (strict)"("DisabledEnum"=T9."Enabled" ("Disabled")) -> ()  [unwired: 2 in, 2 out]
        n204 = property on="ENTER SN" class="Str"("Value"="XXXXX-XX" ("ENTER SN")) -> ()  [unwired: 2 in, 2 out]
        n205 = property on="STEP VARS" class="Clust (strict)"() -> ("Value"=w306:T4)  [unwired: 2 in, 2 out]
        n206 = property on="ENTER OP" class="Str"("Value"="XXXXXX" ("ENTER OP")) -> ()  [unwired: 2 in, 2 out]
        n207 = property on="AP%" class="DigNum (strict)"("Value"=w314) -> ()  [unwired: 2 in, 2 out]
        n208 = property on="T10" class="DigNum (strict)"("Value"=w314) -> ()  [unwired: 2 in, 2 out]
        n209 = property on="RTC" class="DigNum (strict)"("Value"=w314) -> ()  [unwired: 2 in, 2 out]
        n210 = property on="HS" class="DigNum (strict)"("Value"=w314) -> ()  [unwired: 2 in, 2 out]
        n211 = property on="T100" class="DigNum (strict)"("Value"=w314) -> ()  [unwired: 2 in, 2 out]
        n212 = property on="TUBE" class="DigNum (strict)"("Value"=w314) -> ()  [unwired: 2 in, 2 out]
        n213 = Bundle(cluster=w306, "NAME"=w308, "NOTES"=w308, "PARAMS"=w307, "KV  SP"=w307, "KV  RDG"=w307, "MA/IF  SP"=w307, "MA/IF  RDG"=w307, "init BIAS SP"=w307, "init BIAS RDG"=w307, "max Gx"=w307, "TEST"=w307, "min"=w307, "max"=w307, "LIM1"=w307, "LIM2"=w307, "LIM3"=w307, "LIM4"=w307, "data item"=w307, "chain scheds"=w307, "REPEATS"=w307, "STEP NUM"=w307, "EXP s SP"=w307, "EXP s RDG"=w307, "COOL s SP"=w307, "COOL s RDG"=w307, "scans mode"=w307, "init EfDr"=w307, "init EfDr RDG"=w307, "max Tries"=w307, "init DIFF SP"=w307) -> (w310:T4)
        n214 = property on="schd1-30" class="DigNum (strict)"("Value"=w314) -> ()  [unwired: 2 in, 2 out]
        n215 = property on="CURRENT STEP" class="DigNum (strict)"("Value"=w314) -> ()  [unwired: 2 in, 2 out]
        n216 = property on="schd31-60" class="DigNum (strict)"("Value"=w314) -> ()  [unwired: 2 in, 2 out]
        n217 = property on="sched sel Button" class="Bool (strict)"("DisabledEnum"=T9."Disabled and Grayed Out" ("Disabled")) -> ()  [unwired: 2 in, 2 out]
        n218 = property on="Load Tube Button" class="Bool (strict)"("DisabledEnum"=T9."Enabled" ("Disabled")) -> ()  [unwired: 2 in, 2 out]
        n219 = property on="schd61-80" class="DigNum (strict)"("Value"=w314) -> ()  [unwired: 2 in, 2 out]
        n220 = property on="FINAL STEP" class="DigNum (strict)"("Value"=w314) -> ()  [unwired: 2 in, 2 out]
        n221 = property on="FIRST STEP" class="DigNum (strict)"("Value"=w314) -> ()  [unwired: 2 in, 2 out]
        n222 = property on="STEP VARS" class="Clust (strict)"("Value"=w310) -> ()  [unwired: 2 in, 2 out]
        n223 = Initialize Array("..........", 32 ("dimension size"), 2 ("dimension size")) -> (w329:string[][])
        n224 = Initialize Array("0.00000", 32 ("dimension size"), 19 ("dimension size")) -> (w328:string[][])
        n225 = property on="SchedName" class="Str"("Value"="XXXXXXXXXX" ("SchedNum")) -> ()  [unwired: 2 in, 2 out]
        n226 = property on="SchedNum" class="Str"("Value"="XXXXXXXXXX" ("SchedNum")) -> ()  [unwired: 2 in, 2 out]
        n227 = property on="Schedule" class="MCListbox (strict)"() -> ("ItemNames"=w331:string[][])  [unwired: 2 in, 2 out]
        n228 = Replace Array Subset(array=w331, new element #1=w329, index (row) #1=0 ("index"), index (col) #1=0 ("disabled index (col)"), new element #2=w328, index (row) #2=0 ("index"), index (col) #2=2 ("disabled index (col)")) -> (w330:string[][])
        n229 = property on="Schedule" class="MCListbox (strict)"("ItemNames"=w330) -> ()  [unwired: 2 in, 2 out]
      }
      frame "PLC Step Change" {
        n230 = property on="PLC CURRENT STEP" class="DigNum (strict)"() -> ("Value"=w336:u16)  [unwired: 2 in, 2 out]
        n231 = property on="Schedule" class="MCListbox (strict)"() -> ("ItemNames"=w341:string[][])  [unwired: 2 in, 2 out]
        n232 = property on="PLC CURRENT STEP" class="DigNum (strict)"() -> ("Value"=w342:u16)  [unwired: 2 in, 2 out]
        n233 = Decrement(x=w336) -> (x-1=w337:u16)
        n234 = property on="CURRENT STEP" class="DigNum (strict)"("Value"=w342) -> ()  [unwired: 2 in, 2 out]
        n235 = Index Array(array=w341, index (row)=w337) -> (element=w340:string[])  [unwired: 1 in]
        n236 = call "Schedsteptodisplay.vi"("step num"=w336, "step array"=w340) -> ("STEP VARS"=w339:T4)  [unwired: 9 in]
        n237 = property on="STEP VARS" class="Clust (strict)"("Value"=w339) -> ()  [unwired: 2 in, 2 out]
      }
      frame "PROC OK CHECK" {
        n238 = property on="PROC OK" class="Arr (strict)"() -> ("Value"=w347:bool[])  [unwired: 2 in, 2 out]
        n239 = And Array Elements(Boolean array=w347) -> (logical AND=w346:bool)
        n240 = Not(x=w346) -> (.not. x?=w345:bool)
        n241 = property on="PROC NOK" class="Bool (strict)"("Value"=w345) -> ()  [unwired: 2 in, 2 out]
        n242 = case shown="True" w345 {
          tunnel: w344 -> [w349 w351]
          tunnel: [w349 w350] -> w343
          frame False {
            n243 = property on="RUN Button" class="Bool (strict)"("DisabledEnum"=T9."Enabled" ("Disabled")) -> ()  [unwired: 2 in, 2 out]
          }
          frame True {
            n244 = call "Enqueue Message (Single).vi"("Error In"=w351, "Message Position"=Message_Queue_Element_Position."Front", "State Machine Message"=State_Machine_Message."PROC NOK") -> ("Error Out"=w350:errorcluster)  [unwired: 8 in]
          }
        }
      }
      frame "PROC NOK" {
        n245 = property on="RUN Button" class="Bool (strict)"("DisabledEnum"=T9."Disabled and Grayed Out" ("Disabled")) -> ()  [unwired: 2 in, 2 out]
      }
      frame "ALARM CHECK" {
        n246 = property on="ALARMS" class="Arr (strict)"() -> ("Value"=w359:bool[])  [unwired: 2 in, 2 out]
        n247 = Or Array Elements(Boolean array=w359) -> (logical OR=w356:bool)
        n248 = property on="ALARM" class="Bool (strict)"("Value"=w356) -> ()  [unwired: 2 in, 2 out]
        n249 = case shown="True" w356 {
          tunnel: w358 -> [w360 w362]
          tunnel: [w360 w361] -> w357
          frame False {
          }
          frame True {
            n250 = call "Enqueue Message (Single).vi"("Error In"=w362, "Message Position"=Message_Queue_Element_Position."Front", "State Machine Message"=State_Machine_Message."ALARM ACTIVE") -> ("Error Out"=w361:errorcluster)  [unwired: 8 in]
          }
        }
      }
      frame "ALARM ACTIVE" {
        n251 = property on="RUN Button" class="Bool (strict)"("DisabledEnum"=T9."Disabled and Grayed Out" ("Disabled")) -> ()  [unwired: 2 in, 2 out]
      }
      frame "Handle Error" {
        n252 = Variant To Data(type=errorcluster {"status"=FALSE, "code"=0, "source"=""} ("Error In"), Variant=w371) -> (data=w368:errorcluster, error out=w370:errorcluster)  [unwired: 1 in]
        n253 = Merge Errors(w370, w369) -> (w367:errorcluster)
        n254 = call <vilib>:"Simple Error Handler.vi"("error in (no error)"=w368) -> ()  [unwired: 4 in, 5 out]
      }
      frame "Exit" {
        n255 = call "Flush Message Queue.vi"("Error In"=w374) -> ("Error Out"=w373:errorcluster)  [unwired: 9 in, 1 out]
      }
    }
    n256 = call "Enqueue Handle Error Message on Error.vi"("Error In"=w91) -> ("Error Out"=w90:errorcluster)  [unwired: 10 in]
  }
  n257 = Merge Errors(w10, w9) -> (w8:errorcluster)
  n258 = call "Destroy Message Queue.vi"("Error In"=w8) -> ("Error Out"=→"Error Out":errorcluster)  [unwired: 10 in]
  "BADGE NUMBER" <- w14
  "Op Name" <- w14
  "Access" <- u16 0 ("Access")
  "TUBE" <- w3
  "RTC" <- w3
  "HS" <- w3
  "T100" <- w3
  "T10" <- w3
  "AP%" <- w3
  "NAME" <- "XXXXXXXXXX" ("NAME")
  "schd1-30" <- w2
  "schd31-60" <- w2
  "schd61-80" <- w2
  "SchedNum" <- w1
  "SchedName" <- w1
